vi "ScanDelayGetMinMaxCurrScannerFrequency.vi"(8 "error in (no error)":errorcluster, 9 "wait":u32=10, 11 "VISA resource name in":refnum<visa-resource-name>) -> (0 "error out":errorcluster, 2 "value":dbl, 3 "VISA resource name out":refnum<visa-resource-name>, 4 "min":dbl, 5 "max":dbl)   [LabVIEW 2018]
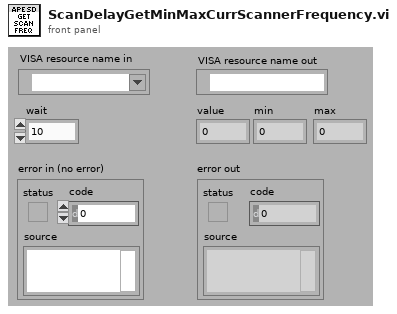
[diagram p1: front panel]
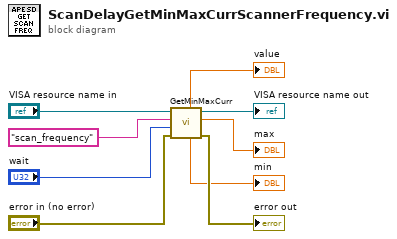
[diagram p0: block diagram]
diagram:
  n1 = call "GetMinMaxCurr.vi"("VISA resource name in"="VISA resource name in", "parameter"="scan_frequency", "wait"="wait", "error in (no error)"="error in (no error)") -> ("value"=→"value":dbl, "MIN"=→"min":dbl, "VISA resource name out"=→"VISA resource name out":refnum<visa-resource-name>, "MAX"=→"max":dbl, "error out"=→"error out":errorcluster)  [unwired: 2 in]
